vi "Get_VI_Reference.vi"(0 "Application_Directory":path, 5 "File_Path":path, 11 "Error_In":errorcluster) -> (4 "VI_Reference":refnum<vi>, 15 "Error_Out":errorcluster)   [LabVIEW 2023]
doc: "Used to get VI reference"
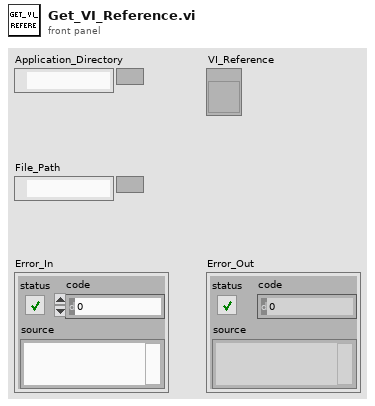
[diagram p1: front panel]
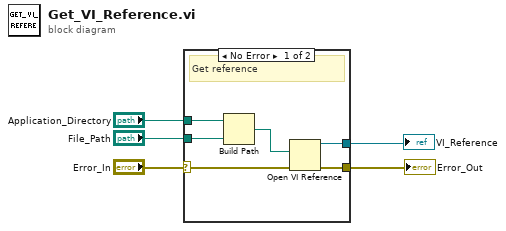
[diagram p0: block diagram]
diagram:
  n1 = case shown="No Error" "Error_In" {
    selector: "Error_In" -> [w9 w12]
    tunnel: [w10 w12] -> w5
    tunnel: "Application_Directory" -> [w8 _]
    tunnel: "File_Path" -> [w7 _]
    tunnel: [w6 _] -> w1
    frame No Error {
      # "Get reference"
      n2 = Build Path(base path=w8, name or relative path=w7) -> (appended path=w11:path)
      n3 = Open VI Reference(vi path=w11, error in (no error)=w9) -> (vi reference=w6:refnum<vi>, error out=w10:errorcluster)  [unwired: 4 in]
    }
    frame Error {
    }
  }
  "Error_Out" <- w5
  "VI_Reference" <- w1
